vi "Write (0D Bool).vi"(8 "error in (no error)":errorcluster, 9 "offset (0)":u64 format="%d bytes", 10 "value":bool, 11 "Pointer in":refnum<class "Pointer.lvclass">) -> (0 "error out":errorcluster, 1 "offset out":u64 format="%d bytes", 2 "value":bool, 3 "Pointer out":refnum<class "Pointer.lvclass">)   [LabVIEW 2017, in "Memory Manager.lvlib" / "Pointer.lvclass"]
doc: "Writes the provided <b>value</b> to the address specified by <b>pointer + offset</b>.\n\n<b>Note:</b> This VI is <b>safe</b>.\n\nSafe means that this function evaluates the size parameter of <b>pointer</b> to ensure that is inbounds of allocated memory before peforming a memory read/write. Reading/writing more data to a pointer than it has allocated can corrupt or crash LabVIEW."
uses:
  Pointer.lvclass
  Pointer.lvclass/Pointer.ctl
  API/Accessors/Get Address.vi
  Protected/Errors.vi
  Protected/Error VIs/Null Pointer.vi
  Protected/Error VIs/Out of Bounds.vi
  API/Accessors/Get Size.vi
  Protected/Error Building/Create Error.vi
  Protected/Error Building/Write Pointer Size.vi
  Protected/Error Building/Get Error Info.vi
  VIs/Write String into Source.vi
  VIs/Write Number into Source.vi
  VIs/VIs for Poly/Write U64 into Source.vi
  VIs/Set Error Source.vi
  VIs/Set Error Code.vi
  VIs/Set Error Status.vi
  Constants/Constants.vi
  Constants/Library Name.vi
  VIs/Create Error Cluster.vi
  VIs/VIs for Poly/Create Error Cluster (256B).vi
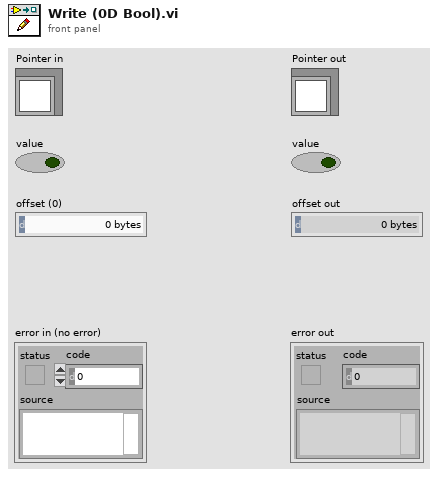
[diagram p1: front panel]
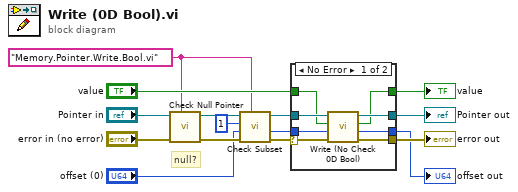
[diagram p0: block diagram]
diagram:
  w5 = "Memory.Pointer.Write.Bool.vi" ("source vi name")
  # "null?"
  n1 = call "Check Null Pointer.vi"("source vi name"=w5, "error in (no error)"="error in (no error)", "Pointer in"="Pointer in") -> ("error out"=w7:errorcluster, "Pointer out"=w6:refnum<class "Pointer.lvclass">)  [unwired: 7 in]
  n2 = call "Check Subset.vi"("source vi name"=w5, "error in (no error)"=w7, "offset (0)"="offset (0)", "length"=u64 1 ("y"), "Pointer in"=w6) -> ("error out"=w14:errorcluster, "offset out"=w3:u64, "Pointer out"=w15:refnum<class "Pointer.lvclass">)  [unwired: 3 in, 1 out]
  n3 = case shown="No Error" w14 {
    selector: w14 -> [w19 w25]
    tunnel: w15 -> [w23 w27]
    tunnel: [w22 w27] -> w10
    tunnel: [w21 w26] -> w11
    tunnel: "value" -> [w20 w26]
    tunnel: [w18 w25] -> w13
    tunnel: w3 -> [w17 w24]
    tunnel: [w16 w24] -> w4
    frame No Error {
      n4 = call "Write (No Check 0D Bool).vi"("error in (no error)"=w19, "offset (0)"=w17, "value"=w20, "Pointer in"=w23) -> ("error out"=w18:errorcluster, "offset out"=w16:u64, "value"=w21:bool, "Pointer out"=w22:refnum<class "Pointer.lvclass">)  [unwired: 4 in]
    }
    frame Error {
    }
  }
  "error out" <- w13
  "Pointer out" <- w10
  "value" <- w11
  "offset out" <- w4
